vi "Parse (Raw Acceleration And Angular Rates).vi"(7 "Message In":string) -> (4 "Raw Accelerometer Vector":sgl[](array[numeric]), 8 "Raw Angular Rate Vector":sgl[](array[numeric]), 15 "Timer":u32)   [LabVIEW 2012, in "MicroStrain 3DM-GXx.lvlib"]
doc: "Parse the data from the 0xC1 message into the Raw Accelerometer Vector (volts) and Raw Angular Rate Vector (volts)."
uses:
  <instrlib>/MicroStrain 3DM-GXx/MicroStrain 3DM-GXx.lvlib
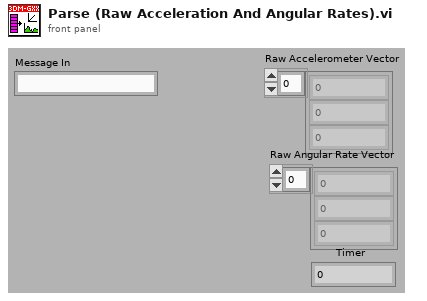
[diagram p1: front panel]
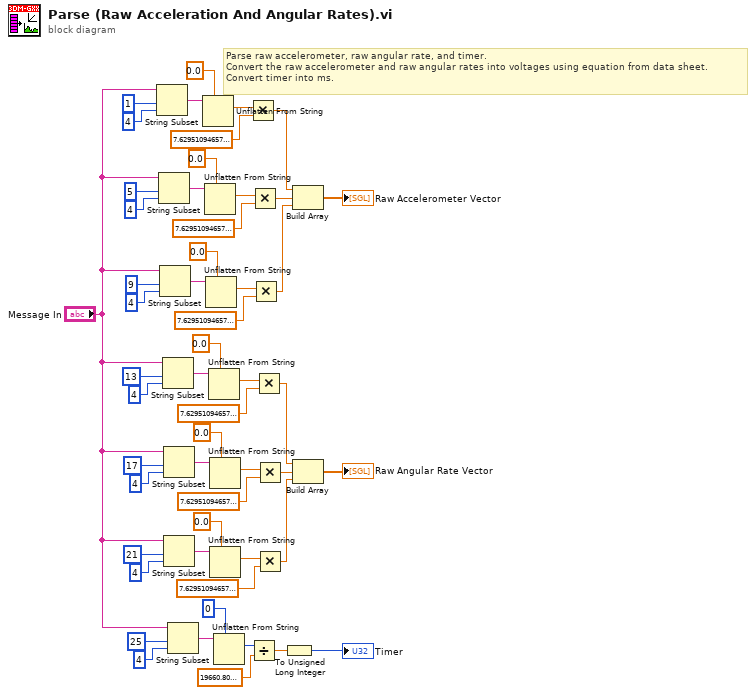
[diagram p0: block diagram]
diagram:
  # "Parse raw accelerometer, raw angular rate, and timer.\nConvert the raw accelerometer and raw angular rates into voltages using equation from data sheet.\nConvert timer into ms."
  n1 = String Subset(string="Message In", offset (0)=1, length (rest)=4 ("length (rest)")) -> (substring=w50:string)
  n2 = String Subset(string="Message In", offset (0)=5, length (rest)=4 ("length (rest)")) -> (substring=w46:string)
  n3 = String Subset(string="Message In", offset (0)=9, length (rest)=4 ("length (rest)")) -> (substring=w42:string)
  n4 = String Subset(string="Message In", offset (0)=13, length (rest)=4 ("length (rest)")) -> (substring=w35:string)
  n5 = String Subset(string="Message In", offset (0)=17, length (rest)=4 ("length (rest)")) -> (substring=w30:string)
  n6 = String Subset(string="Message In", offset (0)=21, length (rest)=4 ("length (rest)")) -> (substring=w27:string)
  n7 = String Subset(string="Message In", offset (0)=25, length (rest)=4 ("length (rest)")) -> (substring=w18:string)
  n8 = Unflatten From String(type=sgl 0.0, binary string=w50) -> (value=w12:sgl)  [unwired: 3 in, 2 out]
  n9 = Unflatten From String(type=sgl 0.0, binary string=w46) -> (value=w10:sgl)  [unwired: 3 in, 2 out]
  n10 = Unflatten From String(type=sgl 0.0, binary string=w42) -> (value=w8:sgl)  [unwired: 3 in, 2 out]
  n11 = Unflatten From String(type=sgl 0.0, binary string=w35) -> (value=w6:sgl)  [unwired: 3 in, 2 out]
  n12 = Unflatten From String(type=sgl 0.0, binary string=w30) -> (value=w3:sgl)  [unwired: 3 in, 2 out]
  n13 = Unflatten From String(type=sgl 0.0, binary string=w27) -> (value=w1:sgl)  [unwired: 3 in, 2 out]
  n14 = Unflatten From String(type=u32 0, binary string=w18) -> (value=w15:u32)  [unwired: 3 in, 2 out]
  n15 = Multiply(x=w12, y=sgl 7.629511e-05 ("x")) -> (x*y=w39:sgl)
  n16 = Divide(x=w15, y=sgl 19660.8) -> (x/y=w14:sgl)
  n17 = Multiply(x=w10, y=sgl 7.629511e-05 ("x")) -> (x*y=w40:sgl)
  n18 = Multiply(x=w8, y=sgl 7.629511e-05 ("x")) -> (x*y=w38:sgl)
  n19 = Multiply(x=w6, y=sgl 7.629511e-05 ("x")) -> (x*y=w23:sgl)
  n20 = Multiply(x=w3, y=sgl 7.629511e-05 ("x")) -> (x*y=w24:sgl)
  n21 = Multiply(x=w1, y=sgl 7.629511e-05 ("x")) -> (x*y=w22:sgl)
  n22 = To Unsigned Long Integer(number=w14) -> (unsigned 32bit integer=→"Timer":u32)
  n23 = Build Array(w39, w40, w38) -> (→"Raw Accelerometer Vector":sgl[])
  n24 = Build Array(w23, w24, w22) -> (→"Raw Angular Rate Vector":sgl[])
